vi "controlRealtimeInputLoopMode.vi"(7 "Set":bool, 8 "error in":errorcluster, 9 "RT Loop in":i32, 10 "axis in":u8, 11 "connection ID":refnum<k5>) -> (0 "error out":errorcluster, 1 "RT Loop out":i32, 2 "axis out":u8, 3 "connection ID":refnum<k5>)   [LabVIEW 2019]
panel:
  in  "Set Command 1":string="com.attocube.amc.rtin.setRealTimeInFeedbackLoopMode"
  in  "Get Command":string="com.attocube.amc.rtin.getRealTimeInFeedbackLoopMode"
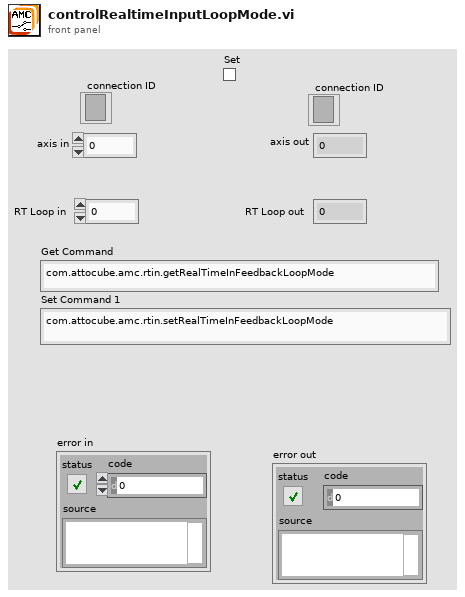
[diagram p1: front panel]
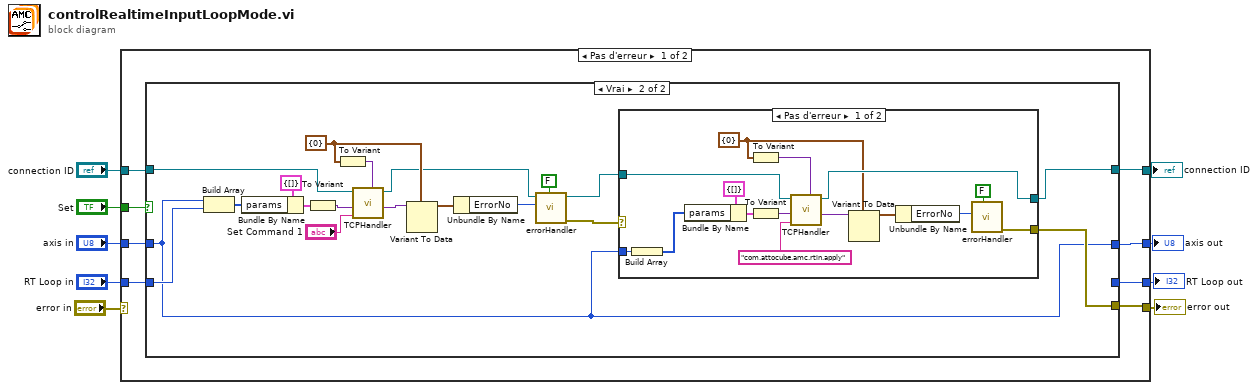
[diagram p0: block diagram]
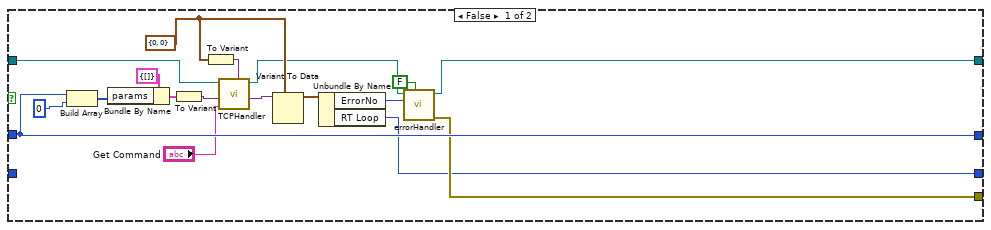
[diagram p2: hidden frame]
diagram:
  n1 = case shown="Pas d'erreur" "error in" {
    selector: "error in" -> [_ w75]
    tunnel: "axis in" -> [w15 w73]
    tunnel: [w10 w75] -> w8
    tunnel: [w12 w73] -> w7
    tunnel: "Set" -> [w16 _]
    tunnel: [w13 w72] -> w5
    tunnel: "connection ID" -> [w17 w72]
    tunnel: "RT Loop in" -> [w14 w74]
    tunnel: [w11 w74] -> w2
    frame No Error {
      n2 = case shown="Vrai" w16 {
        tunnel: [w31 w37] -> w13
        tunnel: w17 -> [w33 w54]
        tunnel: w15 -> [w35 w36]
        tunnel: [w35 w36] -> w12
        tunnel: [w34 w38] -> w10
        tunnel: [w32 _] -> w11
        tunnel: w14 -> [_ w53]
        frame False {
          w21 = cluster{"ErrorNo":i16, "RT Loop":i64} {"ErrorNo"=0, "RT Loop"=0} ("input cluster")
          n3 = Build Array(w35, u8 0 ("element")) -> (w26:u8[])
          n4 = Bundle By Name(cluster=cluster{"params":i16[]} {"params"=[]} ("input cluster"), "params"=w26) -> (w27:cluster{"params":i16[]})
          n5 = To Variant(anything=w27) -> (Variant=w28:variant)
          n6 = To Variant(anything=w21) -> (Variant=w22:variant)
          n7 = call "TCPHandler.vi"("result Types"=w22, "method"="Get Command", "params"=w28, "connection ID"=w33) -> ("result"=w24:variant, "connection ID"=w19:refnum<k5>)  [unwired: 5 in, 1 out]
          n8 = Variant To Data(type=w21, Variant=w24) -> (data=w29:cluster{"ErrorNo":i16, "RT Loop":i64})  [unwired: 1 in, 1 out]
          n9 = Unbundle By Name(w29) -> ("ErrorNo"=w30:i16, "RT Loop"=w32:i64)
          n10 = call "errorHandler.vi"("show popup"=FALSE, "error number"=w30, "connection ID"=w19) -> ("error out"=w34:errorcluster, "connection ID"=w31:refnum<k5>)  [unwired: 7 in]
        }
        frame True {
          w43 = cluster{"ErrorNo":i16} {"ErrorNo"=0} ("input cluster")
          n11 = Build Array(w36, w53) -> (w49:i32[])
          n12 = Bundle By Name(cluster=cluster{"params":i64[]} {"params"=[]} ("input cluster"), "params"=w49) -> (w48:cluster{"params":i64[]})
          n13 = To Variant(anything=w48) -> (Variant=w47:variant)
          n14 = To Variant(anything=w43) -> (Variant=w44:variant)
          n15 = call "TCPHandler.vi"("result Types"=w44, "method"="Set Command 1", "params"=w47, "connection ID"=w54) -> ("result"=w51:variant, "connection ID"=w42:refnum<k5>)  [unwired: 5 in, 1 out]
          n16 = Variant To Data(type=w43, Variant=w51) -> (data=w46:cluster{"ErrorNo":i16})  [unwired: 1 in, 1 out]
          n17 = Unbundle By Name(w46) -> ("ErrorNo"=w45:i16)
          n18 = call "errorHandler.vi"("show popup"=FALSE, "error number"=w45, "connection ID"=w42) -> ("error out"=w40:errorcluster, "connection ID"=w39:refnum<k5>)  [unwired: 7 in]
          n19 = case shown="Pas d'erreur" w40 {
            selector: w40 -> [_ w71]
            tunnel: w39 -> [w69 w70]
            tunnel: [w63 w71] -> w38
            tunnel: [w62 w70] -> w37
            tunnel: w36 -> [w57 _]
            frame No Error {
              w55 = cluster{"ErrorNo":i16} {"ErrorNo"=0} ("input cluster")
              n20 = Build Array(w57) -> (w61:u8[])
              n21 = Bundle By Name(cluster=cluster{"params":i64[]} {"params"=[]} ("input cluster"), "params"=w61) -> (w59:cluster{"params":i64[]})
              n22 = To Variant(anything=w55) -> (Variant=w56:variant)
              n23 = To Variant(anything=w59) -> (Variant=w58:variant)
              n24 = call "TCPHandler.vi"("result Types"=w56, "method"="com.attocube.amc.rtin.apply" ("Set Command 2"), "params"=w58, "connection ID"=w69) -> ("result"=w66:variant, "connection ID"=w62:refnum<k5>)  [unwired: 5 in, 1 out]
              n25 = Variant To Data(type=w55, Variant=w66) -> (data=w67:cluster{"ErrorNo":i16})  [unwired: 1 in, 1 out]
              n26 = Unbundle By Name(w67) -> ("ErrorNo"=w65:i16)
              n27 = call "errorHandler.vi"("show popup"=FALSE, "error number"=w65) -> ("error out"=w63:errorcluster)  [unwired: 8 in, 1 out]
            }
            frame Error {
            }
          }
        }
      }
    }
    frame Error {
    }
  }
  "error out" <- w8
  "axis out" <- w7
  "connection ID" <- w5
  "RT Loop out" <- w2
